vi "Set Probe Params by Index.vi"(9 "Index":i32, 11 "Probe Cfg Params":T1 {"Sensor Block"."SensorCfgParams Array"."CalibrCoefArray" format="%#.12g"}) -> ()   [LabVIEW 2015, in "Tool Cfg.lvlib"]
uses:
  Tool Cfg.lvlib
  _ProbeConfigParams Cluster--typedef.ctl
  _Sensor Block Cluster--typedef.ctl
  _SensorConfigParams Cluster--typedef.ctl
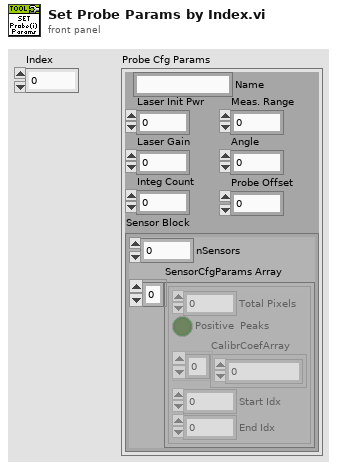
[diagram p1: front panel]
types:
  T1 = typedef "Tool Cfg.lvlib/_ProbeConfigParams Cluster--typedef.ctl" = cluster{"Name":string, "Laser Init Pwr":u16, "Laser Gain":u8, "Integ Count":u16, "Meas. Range":sgl, "Angle":sgl, "Probe Offset":sgl, "Sensor Block":T2}
  T2 = typedef "Tool Cfg.lvlib/_Sensor Block Cluster--typedef.ctl" = cluster{"nSensors":u16, "SensorCfgParams Array":T3[]}
  T3 = typedef "Tool Cfg.lvlib/_SensorConfigParams Cluster--typedef.ctl" = cluster{"Total Pixels":u16, "Positive  Peaks":bool, "CalibrCoefArray":dbl[], "Start Idx":u16, "End Idx":u16}
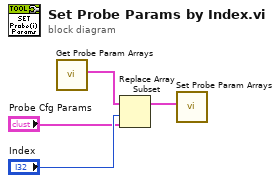
[diagram p0: block diagram]
diagram:
  n1 = call "Get Probe Param Arrays.vi"() -> ("Probe Block.Probe Param Array"=w2:T1[])  [unwired: 10 in, 1 out]
  n2 = Replace Array Subset(array=w2, new element="Probe Cfg Params", index="Index") -> (w1:T1[])
  n3 = call "Set Probe Param Arrays.vi"("Probe Param Array"=w1) -> ()  [unwired: 11 in]
